vi "Combine Particles.vi"(11 "Good particles in":T1(array[cluster])) -> (0 "Unpaired particles":T1(array[cluster]), 3 "Unmeasured Targets":T2[](array[typedef]))   [LabVIEW 2015]
uses:
  Vision Tote Data.ctl
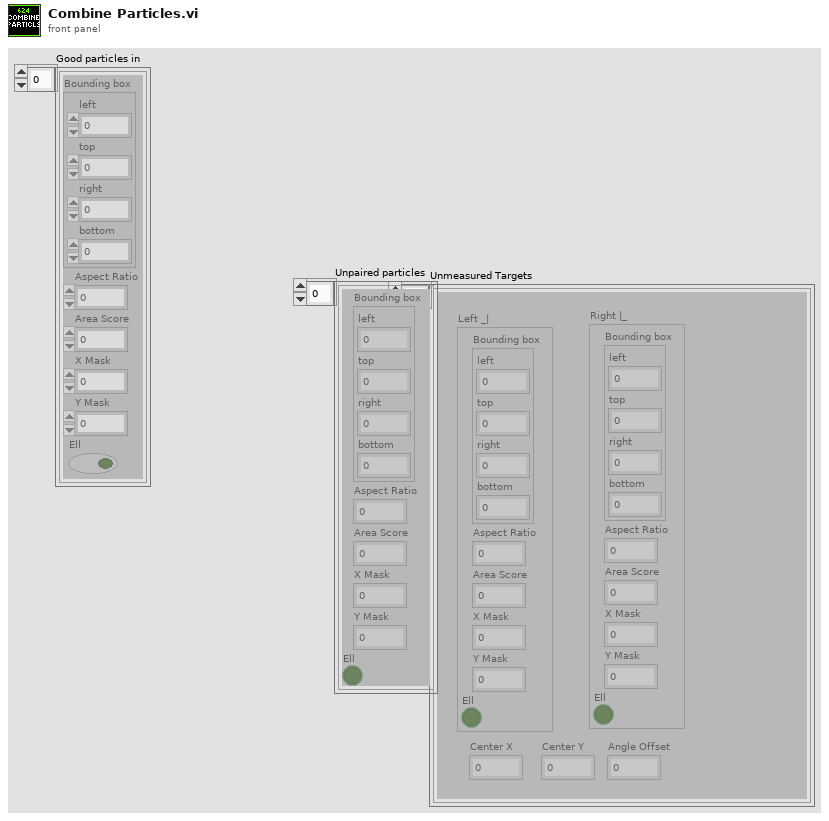
[diagram p1: front panel]
types:
  T1 = cluster{"Bounding box":cluster{"left":dbl, "top":dbl, "right":dbl, "bottom":dbl}, "Aspect Ratio":dbl, "Area Score":dbl, "X Mask":dbl, "Y Mask":dbl, "Ell":bool}[]
  T2 = typedef "Vision Tote Data.ctl" = cluster{"Left _|":cluster{"Bounding box":cluster{"left":dbl, "top":dbl, "right":dbl, "bottom":dbl}, "Aspect Ratio":dbl, "Area Score":dbl, "X Mask":dbl, "Y Mask":dbl, "Ell":bool}, "Right |_":cluster{"Bounding box":cluster{"left":dbl, "top":dbl, "right":dbl, "bottom":dbl}, "Aspect Ratio":dbl, "Area Score":dbl, "X Mask":dbl, "Y Mask":dbl, "Ell":bool}, "Center X":dbl, "Center Y":dbl, "Angle Offset":dbl}
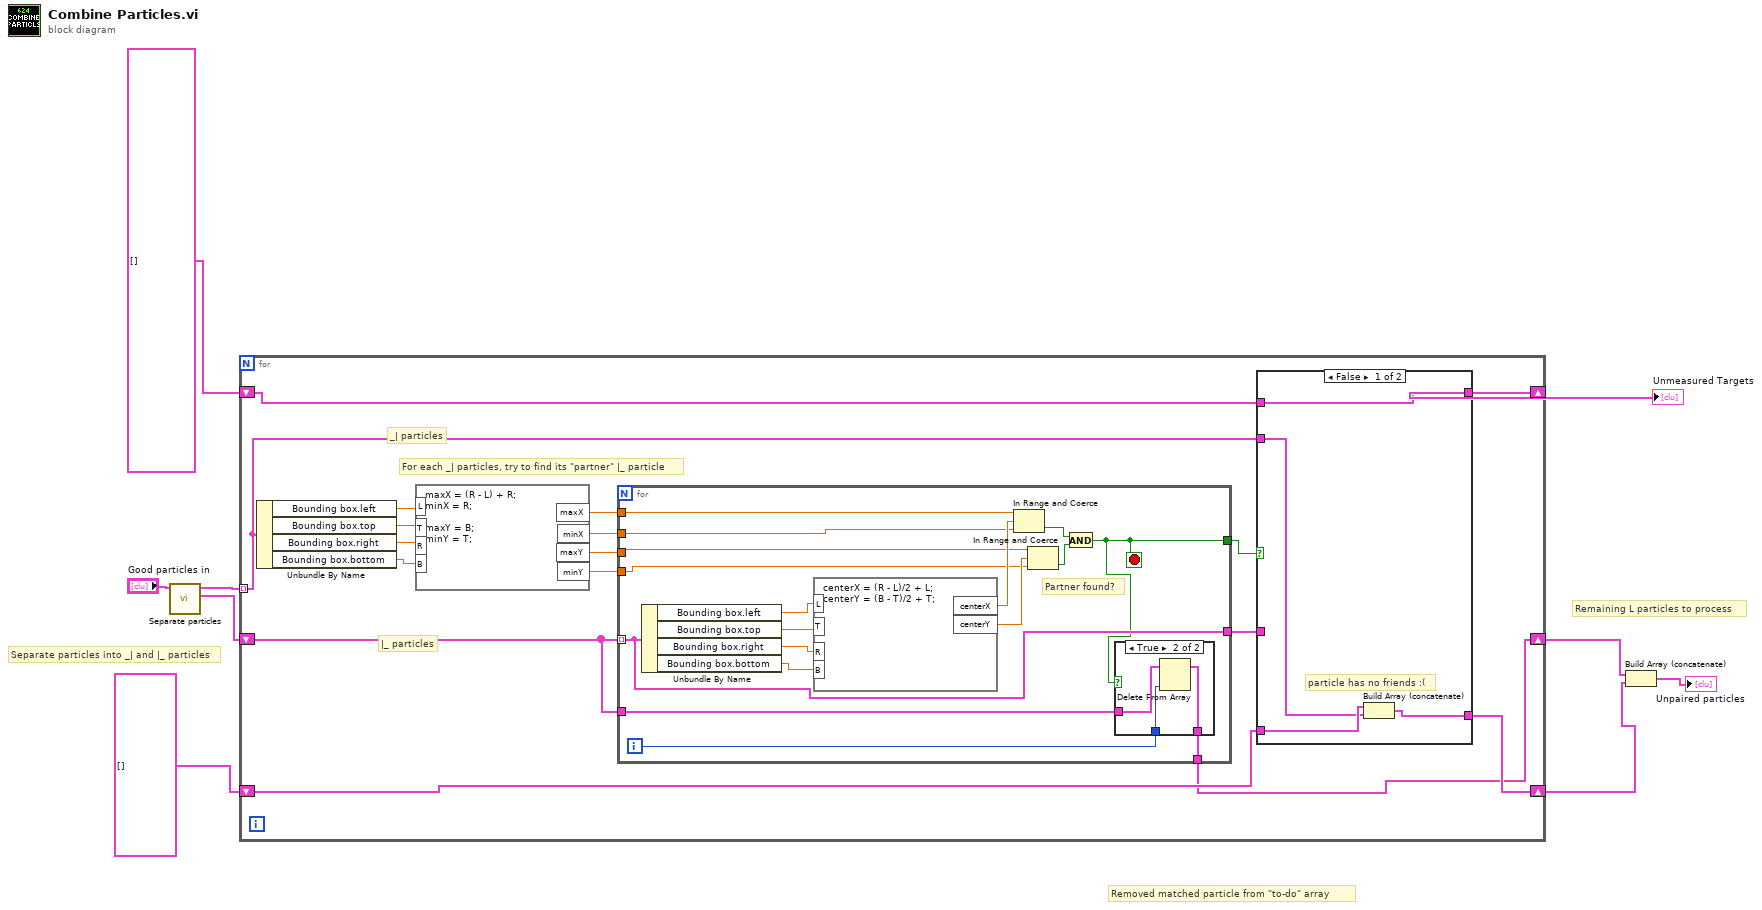
[diagram p0: block diagram]
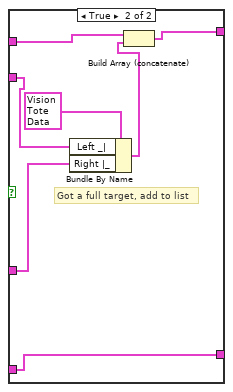
[diagram p2: hidden frame]
diagram:
  # "Removed matched particle from \"to-do\" array"
  # "Remaining L particles to process"
  # "Separate particles into _| and |_ particles"
  n1 = call "Separate particles.vi"("Good particles in 3"="Good particles in") -> ("|_ particles"=w7:T1, "_| particles"=w8:T1)  [unwired: 9 in]
  n2 = for {
    tunnel: w8 -> [w16] mode=indexing
    shift-right: [w15] -> w5
    shift-left: T2[] [] ("appended array") -> [w14]
    shift-right: [w12] -> w2
    shift-left: T1 [] ("Unpaired particles") -> [w13]
    shift-right: [w10] -> w3
    shift-left: w7 -> [w11]
    # "|_ particles"
    # "_| particles"
    # "For each _| particles, try to find its \"partner\" |_ particle"
    n3 = Unbundle By Name(w16) -> ("Bounding box.left"=w26:dbl, "Bounding box.top"=w25:dbl, "Bounding box.right"=w24:dbl, "Bounding box.bottom"=w23:dbl)
    n4 = formula code="maxX = (R - L) + R;\nminX = R;\n\nmaxY = B;\nminY = T;"("L"=w26, "T"=w25, "R"=w24, "B"=w23) -> ("maxX"=w22:dbl, "minX"=w21:dbl, "maxY"=w20:dbl, "minY"=w19:dbl)
    n5 = for {
      tunnel: w11 -> [w42] mode=indexing
      tunnel: w22 -> [w49]
      tunnel: w21 -> [w48]
      tunnel: w20 -> [w46]
      tunnel: w19 -> [w45]
      tunnel: [w40] -> w18
      tunnel: [w42] -> w17
      tunnel: w11 -> [w41]
      tunnel: [w38] -> w10
      i -> [w39]
      stop <- w40 stop-if-true
      # "Partner found?"
      n6 = Unbundle By Name(w42) -> ("Bounding box.left"=w54:dbl, "Bounding box.top"=w53:dbl, "Bounding box.right"=w52:dbl, "Bounding box.bottom"=w51:dbl)
      n7 = formula code="centerX = (R - L)/2 + L;\ncenterY = (B - T)/2 + T;"("L"=w54, "T"=w53, "R"=w52, "B"=w51) -> ("centerX"=w50:dbl, "centerY"=w47:dbl)
      n8 = In Range and Coerce(upper limit=w49, x=w50, lower limit=w48) -> (In Range?=w43:bool)  [unwired: 1 out]
      n9 = In Range and Coerce(upper limit=w46, x=w47, lower limit=w45) -> (In Range?=w44:bool)  [unwired: 1 out]
      n10 = And(x=w43, y=w44) -> (x .and. y?=w40:bool)
      n11 = case shown="True" w40 {
        tunnel: w41 -> [w55 w58]
        tunnel: w39 -> [_ w57]
        tunnel: [w55 w56] -> w38
        frame False {
        }
        frame True {
          n12 = Delete From Array(array=w58, index=w57) -> (array with subset deleted=w56:T1)  [unwired: 1 in, 1 out]
        }
      }
    }
    n13 = case shown="False" w18 {
      tunnel: w17 -> [_ w35]
      tunnel: w16 -> [w28 w36]
      tunnel: [w30 w32] -> w15
      tunnel: w14 -> [w30 w34]
      tunnel: w13 -> [w29 w31]
      tunnel: [w27 w31] -> w12
      frame False {
        # "particle has no friends :("
        n14 = Build Array (concatenate)(w29, w28) -> (w27:T1)
      }
      frame True {
        # "Got a full target, add to list"
        n15 = Bundle By Name(cluster=T2 {"Left _|"={"Bounding box"={"left"=305.0, "top"=258.0, "right"=432.0, "bottom"=368.0}, "Aspect Ratio"=84.54545454545455, "Area Score"=96.6320687186829, "X Mask"=100.0, "Y Mask"=98.18181818181819, "Ell"=TRUE}, "Right |_"={"Bounding box"={"left"=305.0, "top"=258.0, "right"=432.0, "bottom"=368.0}, "Aspect Ratio"=84.54545454545455, "Area Score"=96.6320687186829, "X Mask"=100.0, "Y Mask"=98.18181818181819, "Ell"=TRUE}, "Center X"=0.0, "Center Y"=0.0, "Angle Offset"=0.0} ("Vision Tote Data"), "Left _|"=w36, "Right |_"=w35) -> (w33:T2)
        n16 = Build Array (concatenate)(w34, w33) -> (w32:T2[])
      }
    }
  }
  "Unmeasured Targets" <- w5
  n17 = Build Array (concatenate)(w3, w2) -> (→"Unpaired particles":T1)
